vi "save xml for traverse.vi"(8 "error in":errorcluster caption="错误输入（无错误）", 10 "Data in":T1, 11 "PanelRootNode 输入":refnum<class "PanelRootNode.lvclass"> caption="DNL_LabVIEW Object in") -> (0 "error out":errorcluster caption="错误输出", 2 "Data out":T1, 3 "PanelRootNode 输出":refnum<class "PanelRootNode.lvclass"> caption="DNL_LabVIEW Object out")   [LabVIEW 2016, in "PanelRootNode.lvclass"]
uses:
  PanelRootNode.lvclass
  C:/Users/CL/Desktop/ZcDAQprj0811/ZcDAQprj/Modules/DAQ-Display/PanelSplitToolkit/PanelLinkNode/PanelLinkNode.lvclass
  PanelLinkNode/PanelLinkNode.lvclass/PanelLinkNode.ctl
  <resource>/objmgr/DOMUserDefRef.rc
  PanelLinkNode/PanelLinkNode.lvclass
  <vilib>/xml/NI_XML.lvlib
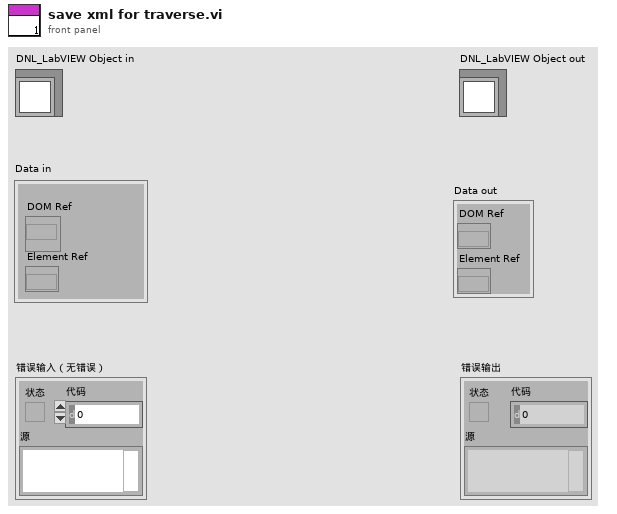
[diagram p1: front panel]
types:
  T1 = cluster{"DOM Ref":refnum<k20>, "Element Ref":refnum<k20>}
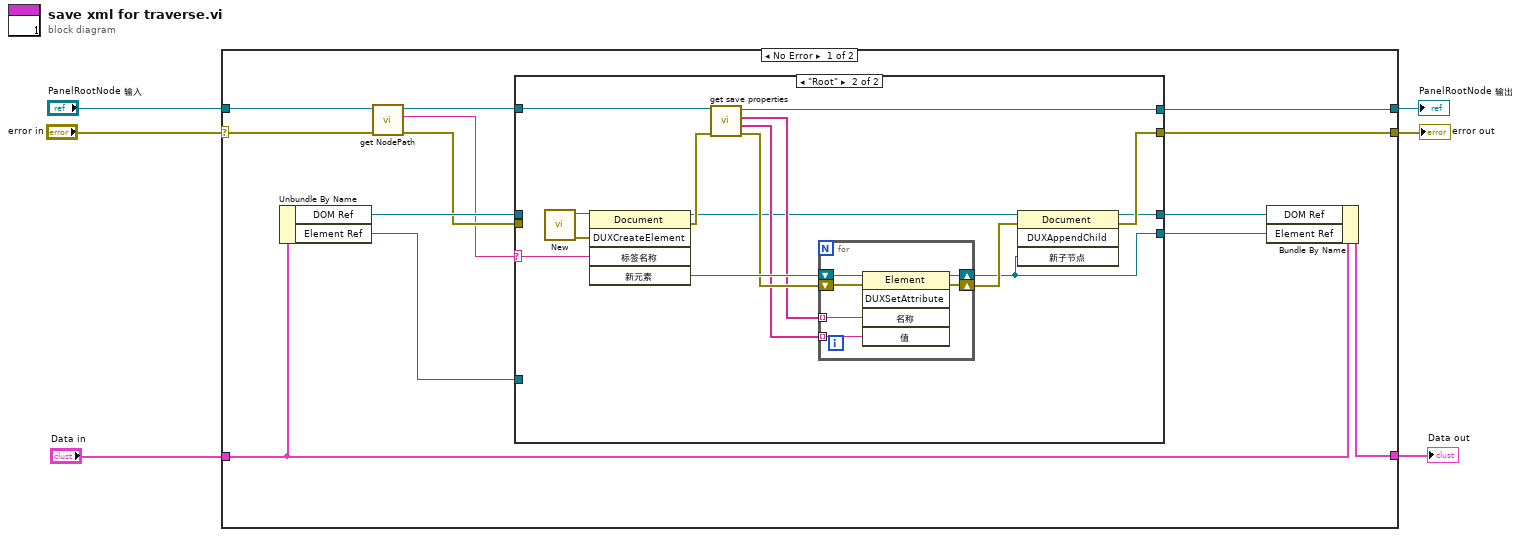
[diagram p0: block diagram]
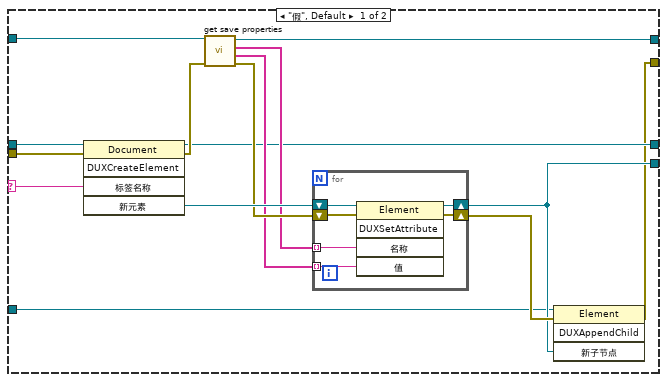
[diagram p2: hidden frame]
diagram:
  n1 = case shown="No Error" "error in" {
    selector: "error in" -> [w11 w64]
    tunnel: [w12 w64] -> w5
    tunnel: [w17 w63] -> w3
    tunnel: "PanelRootNode 输入" -> [w19 w63]
    tunnel: "Data in" -> [w16 w62]
    tunnel: [w13 w62] -> w1
    frame No Error {
      n2 = Unbundle By Name(w16) -> ("DOM Ref"=w10:refnum<k20>, "Element Ref"=w9:refnum<k20>)
      n3 = call "get NodePath.vi"("error in (no error)"=w11, "PanelLinkNode输入"=w19) -> ("error out"=w8:errorcluster, "NodePath"=w7:string, "PanelLinkNode输出"=w18:refnum<class "PanelRootNode.lvclass">)  [unwired: 7 in]
      n4 = case shown="\"Root\"" w7 {
        selector: w7 -> [w20 w43]
        tunnel: w18 -> [w33 w54]
        tunnel: [w32 w53] -> w17
        tunnel: [w26 w44] -> w15
        tunnel: [w25 w47] -> w14
        tunnel: [w24 w46] -> w12
        tunnel: w10 -> [w23 _]
        tunnel: w9 -> [w22 _]
        tunnel: w8 -> [w21 _]
        frame "假", Default {
          n5 = invoke on="调用节点" class="Document" method="DUXCreateElement"(reference=w23, error in=w21, "标签名称"=w20) -> (reference out=w26:refnum<k20>, error out=w31:errorcluster, "新元素"=w34:refnum<k20>)  [unwired: 2 in, 2 out]
          n6 = call-dynamic "get save properties.vi"("error in"=w31, "PanelRootNode 输入"=w33) -> ("error out"=w30:errorcluster, "Values"=w28:string[], "Names"=w29:string[], "PanelRootNode 输出"=w32:refnum<class "PanelRootNode.lvclass">)  [unwired: 6 in]
          n7 = for {
            tunnel: w29 -> [w38] mode=indexing
            tunnel: w28 -> [w37] mode=indexing
            shift-right: [w36] -> w25
            shift-left: w34 -> [w40]
            shift-right: [w35] -> w27
            shift-left: w30 -> [w39]
            n8 = invoke on="调用节点" class="Element" method="DUXSetAttribute"(reference=w40, error in=w39, "名称"=w38, "值"=w37) -> (reference out=w36:refnum<k20>, error out=w35:errorcluster)  [unwired: 1 in, 3 out]
          }
          n9 = invoke on="调用节点" class="Element" method="DUXAppendChild"(reference=w22, error in=w27, "新子节点"=w25) -> (error out=w24:errorcluster)  [unwired: 1 in, 3 out]
        }
        frame "Root" {
          n10 = call <vilib>:"New.vi"() -> ("error out"=w41:errorcluster, "DOM document out"=w42:refnum<k20>)  [unwired: 8 in]
          n11 = invoke on="调用节点" class="Document" method="DUXCreateElement"(reference=w42, error in=w41, "标签名称"=w43) -> (reference out=w45:refnum<k20>, error out=w52:errorcluster, "新元素"=w55:refnum<k20>)  [unwired: 2 in, 2 out]
          n12 = call-dynamic "get save properties.vi"("error in"=w52, "PanelRootNode 输入"=w54) -> ("error out"=w51:errorcluster, "Values"=w49:string[], "Names"=w50:string[], "PanelRootNode 输出"=w53:refnum<class "PanelRootNode.lvclass">)  [unwired: 6 in]
          n13 = for {
            tunnel: w50 -> [w59] mode=indexing
            tunnel: w49 -> [w58] mode=indexing
            shift-right: [w57] -> w47
            shift-left: w55 -> [w61]
            shift-right: [w56] -> w48
            shift-left: w51 -> [w60]
            n14 = invoke on="调用节点" class="Element" method="DUXSetAttribute"(reference=w61, error in=w60, "名称"=w59, "值"=w58) -> (reference out=w57:refnum<k20>, error out=w56:errorcluster)  [unwired: 1 in, 3 out]
          }
          n15 = invoke on="调用节点" class="Document" method="DUXAppendChild"(reference=w45, error in=w48, "新子节点"=w47) -> (reference out=w44:refnum<k20>, error out=w46:errorcluster)  [unwired: 1 in, 2 out]
        }
      }
      n16 = Bundle By Name(cluster=w16, "DOM Ref"=w15, "Element Ref"=w14) -> (w13:T1)
    }
    frame Error {
    }
  }
  "error out" <- w5
  "PanelRootNode 输出" <- w3
  "Data out" <- w1
